vi "StandardScaler.vi"(8 "error in (no error)":errorcluster caption="entrée d'erreur (pas d'erreur)", 11 "StandardScaler":T1={"copy"=TRUE, "with_mean"=TRUE, "with_std"=TRUE}) -> (0 "error out":errorcluster, 3 "StandardScaler.lvclass":refnum<class "StandardScaler.lvclass">)   [LabVIEW 2020]
doc: "Standardize features by removing the mean and scaling to unit variance\n\nThe standard score of a sample x is calculated as:\n\nz = (x - u) / s\n\nwhere u is the mean of the training samples or zero if with_mean=False, and s is the standard deviation of the training samples or one if with_std=False.\n\nCentering and scaling happen independently on each feature by computing the relevant statistics on the samples in the training set. Mean and standard deviation are then stored to be used on later data using transform.\n\nStandardization of a dataset is a common requirement for many machine learning estimators: they might behave badly if the individual features do not more or less look like standard normally distributed data (e.g. Gaussian with 0 mean and unit variance).\n\nFor instance many elements used in the objective function of a learning algorithm (such as the RBF kernel of Support Vector Machines or the L1 and L2 regularizers of linear models) assume that all features are centered around 0 and have variance in the same order. If a feature has a variance that is orders of magnitude larger that others, it might dominate the objective function and make the estimator unable to learn from other features correctly as expected.\n\nThis scaler can also be applied to sparse CSR or CSC matrices by passing with_mean=False to avoid breaking the sparsity structure of the data.\n\n\nParameters : \n\n- copy : boolean, optional, default True\nIf False, try to avoid a copy and do inplace scaling instead. This is not guaranteed to always work inplace; e.g. if the data is not a NumPy array or scipy.sparse CSR matrix, a copy may still be returned.\n\n- with_mean : boolean, True by default\nIf True, center the data before scaling. This does not work (and will raise an exception) when attempted on sparse matrices, because centering them entails building a dense matrix which in common use cases is likely to be too large to fit in memory.\n\n- with_std : boolean, True by default\nIf True, scale the data to unit variance (or equivalently, unit standard deviation).\n\n\n\nMethods : \n\n- Fit : Compute the mean and std to be used for later scaling.\n\nParameters :\n\nX : {array-like, sparse matrix}, shape [n_samples, n_features]\nThe data used to compute the mean and standard deviation used for later scaling along the features axis.\n\ny : Ignored\n\n\n- Fit Transform : Fit to data, then transform it. Fits transformer to X and y with optional parameters fit_params and returns a transformed version of X.\n\nParameters : \n\nX : {array-like, sparse matrix, dataframe} of shape (n_samples, n_features)\n\ny : ndarray of shape (n_samples,), default=None\nTarget values.\n\nReturns : \n\nX_new : ndarray array of shape (n_samples, n_features_new)\nTransformed array.\n\n\n- Transform : Perform standardization by centering and scaling\n\nParameters : \n\nX : array-like, shape [n_samples, n_features]\nThe data used to scale along the features axis."
uses:
  StandardScaler.lvclass
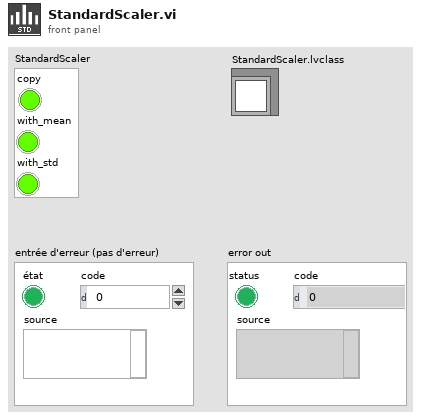
[diagram p1: front panel]
types:
  T1 = cluster{"copy":bool, "with_mean":bool, "with_std":bool}
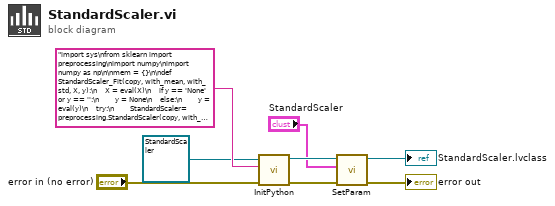
[diagram p0: block diagram]
diagram:
  n1 = call-dynamic "InitPython.vi"("error in (no error)"="error in (no error)", "Python Instruction"="import sys\nfrom sklearn import preprocessing\nimport numpy\nimport numpy as np\n\nmem = {}\n\ndef StandardScaler_Fit(copy, with_mean, with_std, X, y):\n    X = eval(X)\n    if y == 'None' or y == '':\n        y = None\n    else:\n        y = eval(y)\n    try:\n        StandardScaler= preprocessing.StandardScaler(copy, with_mean, with_std).fit(X, y)\n        mem['FitStandardScaler'] = StandardScaler\n        return str('OK')\n    except:\n        erreur = sys.exc_info()\n        typerr = u\"%s\" % (erreur[0])\n        typerr = typerr[typerr.find(\"'\")+1:typerr.rfind(\"'\")]\n        msgerr = u\"%s\" % (erreur[1])\n        message = str('/!\\\\ {0} : {1}'. format(typerr,msgerr))\n        return message \n    \ndef StandardScaler_FitTransform(copy, with_mean, with_std, X, y):\n    X = eval(X)\n    if y == 'None' or y == '':\n        y = None\n    else:\n        y = eval(y)\n    try:\n        StandardScaler = preprocessing.StandardScaler(copy, with_mean, with_std).fit_transform(X, y)\n        dtype = type(StandardScaler)\n        if dtype == numpy.ndarray:\n            StandardScaler = StandardScaler.tolist()\n            return str(StandardScaler) \n        else:\n            Mat = StandardScaler.tocoo()\n            return str(list(zip(Mat.row, Mat.col, Mat.data)))\n    except:\n        erreur = sys.exc_info()\n        typerr = u\"%s\" % (erreur[0])\n        typerr = typerr[typerr.find(\"'\")+1:typerr.rfind(\"'\")]\n        msgerr = u\"%s\" % (erreur[1])\n        message = str('/!\\\\ {0} : {1}'. format(typerr,msgerr))\n        return message \n\ndef StandardScaler_Transform(copy, with_mean, with_std, X, y):\n    X = eval(X)\n    if y == 'None' or y == '':\n        y = None\n    else:\n        y = eval(y)\n    try:\n        StandardScaler = mem['FitStandardScaler'].transform(X)\n        dtype = type(StandardScaler)\n        if dtype == numpy.ndarray:\n            StandardScaler = StandardScaler.tolist()\n            return str(StandardScaler) \n        else:\n            Mat = StandardScaler.tocoo()\n            return str(list(zip(Mat.row, Mat.col, Mat.data)))\n    except:\n        erreur = sys.exc_info()\n        typerr = u\"%s\" % (erreur[0])\n        typerr = typerr[typerr.find(\"'\")+1:typerr.rfind(\"'\")]\n        msgerr = u\"%s\" % (erreur[1])\n        message = str('/!\\\\ {0} : {1}'. format(typerr,msgerr))\n        return message\n    \ndef StandardScaler_Partial_Fit(copy, with_mean, with_std, X, y):\n    X = eval(X)\n    if y == 'None' or y == '':\n        y = None\n    else:\n        y = eval(y)\n    try:\n        StandardScaler = preprocessing.StandardScaler(copy, with_mean, with_std).partial_fit(X, y)\n        mem['FitStandardScaler'] = StandardScaler\n        return str('OK')\n    except:\n        erreur = sys.exc_info()\n        typerr = u\"%s\" % (erreur[0])\n        typerr = typerr[typerr.find(\"'\")+1:typerr.rfind(\"'\")]\n        msgerr = u\"%s\" % (erreur[1])\n        message = str('/!\\\\ {0} : {1}'. format(typerr,msgerr))\n        return message", "Scikit-learn en entrée"=refnum<class "StandardScaler.lvclass"> refnum ("StandardScaler.lvclass")) -> ("error out"=w4:errorcluster, "Scikit-learn en sortie"=w5:refnum<class "StandardScaler.lvclass">)  [unwired: 7 in]
  n2 = call-dynamic "SetParam.vi"("error in (no error)"=w4, "StandardScaler"="StandardScaler", "StandardScaler.lvclass"=w5) -> ("error out"=→"error out":errorcluster, "StandardScaler.lvclass"=→"StandardScaler.lvclass":refnum<class "StandardScaler.lvclass">)  [unwired: 7 in]
